vi "Configure Serial Bus.vi"   [LabVIEW 2010, in "Agilent 2000 3000 X-Series.lvlib"]
doc: "Configures the settings of serial bus."
uses:
  <instrlib>/Agilent 2000 3000 X-Series/Agilent 2000 3000 X-Series.lvlib
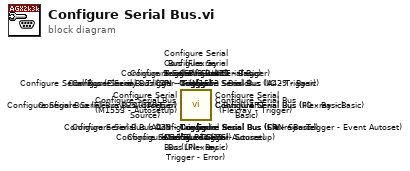
[diagram p0: block diagram]
diagram:
  n1 = call <instrlib>:"Configure Serial Bus (M1553 - Trigger).vi"() -> ()  [unwired: 14 in, 2 out]
  n2 = call <instrlib>:"Configure Serial Bus (M1553 - Basic).vi"() -> ()  [unwired: 14 in, 2 out]
  n3 = call <instrlib>:"Configure Serial Bus (M1553 - Autosetup).vi"() -> ()  [unwired: 14 in, 2 out]
  n4 = call <instrlib>:"Configure Serial Bus (Flexray - Trigger).vi"() -> ()  [unwired: 14 in, 2 out]
  n5 = call <instrlib>:"Configure Serial Bus (Flexray - Trigger - Frame).vi"() -> ()  [unwired: 14 in, 2 out]
  n6 = call <instrlib>:"Configure Serial Bus (Flexray - Trigger - Event).vi"() -> ()  [unwired: 14 in, 2 out]
  n7 = call <instrlib>:"Configure Serial Bus (Flexray - Trigger - Event Autoset).vi"() -> ()  [unwired: 14 in, 2 out]
  n8 = call <instrlib>:"Configure Serial Bus (Flexray - Trigger - Error).vi"() -> ()  [unwired: 14 in, 2 out]
  n9 = call <instrlib>:"Configure Serial Bus (Flexray - Basic).vi"() -> ()  [unwired: 14 in, 2 out]
  n10 = call <instrlib>:"Configure Serial Bus (Flexray - Autosetup).vi"() -> ()  [unwired: 14 in, 2 out]
  n11 = call <instrlib>:"Configure Serial Bus (A429 - Trigger).vi"() -> ()  [unwired: 14 in, 2 out]
  n12 = call <instrlib>:"Configure Serial Bus (A429 - Basic).vi"() -> ()  [unwired: 14 in, 2 out]
  n13 = call <instrlib>:"Configure Serial Bus (A429 - Autosetup).vi"() -> ()  [unwired: 14 in, 2 out]
  n14 = call <instrlib>:"Configure Serial Bus (UART - Trigger).vi"() -> ()  [unwired: 14 in, 2 out]
  n15 = call <instrlib>:"Configure Serial Bus (UART - Source).vi"() -> ()  [unwired: 14 in, 2 out]
  n16 = call <instrlib>:"Configure Serial Bus (UART - Basic).vi"() -> ()  [unwired: 14 in, 2 out]
  n17 = call <instrlib>:"Configure Serial Bus (SPI - Trigger).vi"() -> ()  [unwired: 14 in, 2 out]
  n18 = call <instrlib>:"Configure Serial Bus (SPI - Source).vi"() -> ()  [unwired: 14 in, 2 out]
  n19 = call <instrlib>:"Configure Serial Bus (SPI - Basic).vi"() -> ()  [unwired: 14 in, 2 out]
  n20 = call <instrlib>:"Configure Serial Bus (LIN - Trigger).vi"() -> ()  [unwired: 14 in, 2 out]
  n21 = call <instrlib>:"Configure Serial Bus (LIN - Basic).vi"() -> ()  [unwired: 14 in, 2 out]
  n22 = call <instrlib>:"Configure Serial Bus (IIC - Trigger).vi"() -> ()  [unwired: 14 in, 2 out]
  n23 = call <instrlib>:"Configure Serial Bus (IIC - Basic).vi"() -> ()  [unwired: 14 in, 2 out]
  n24 = call <instrlib>:"Configure Serial Bus (I2S - Trigger).vi"() -> ()  [unwired: 14 in, 2 out]
  n25 = call <instrlib>:"Configure Serial Bus (I2S - Source).vi"() -> ()  [unwired: 14 in, 2 out]
  n26 = call <instrlib>:"Configure Serial Bus (I2S - Basic).vi"() -> ()  [unwired: 14 in, 2 out]
  n27 = call <instrlib>:"Configure Serial Bus (CAN - Trigger).vi"() -> ()  [unwired: 14 in, 2 out]
  n28 = call <instrlib>:"Configure Serial Bus (CAN - Basic).vi"() -> ()  [unwired: 14 in, 2 out]
